vi "CSGaussmeter.setCTemp.vi"(0 "i ref in":refnum<vi>, 7 "CTemp":bool, 11 "error in (no error)":errorcluster) -> (4 "i ref out":refnum<vi>, 15 "error out":errorcluster)   [LabVIEW 2014, in "CSGaussmeter.lvlib"]
doc: "This VI sets the Temp. Correction ON or OFF. \n\nDurch dieses VI kann die Temperaturkorrektur an oder abgeschaltet werden. Die Temperaturkorrektur korrigiert die Temperaturabhängigkeit der Sondenempfindlichkeit und der Offsetspannung."
uses:
  CSGaussmeter.lvlib
  CS_Core/CSObj/CSObj.lvlib
  CSlibraries/UtilityLib/UtilityLib.lvlib
  instr.lib/FH_55/FH 55.lvlib
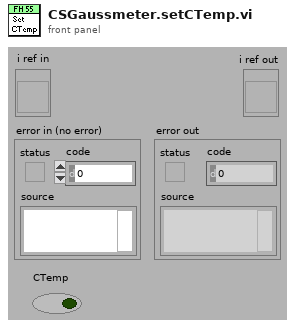
[diagram p1: front panel]
types:
  T1 = typedef "CSGaussmeter.lvlib/CSGaussmeter.i attribute.ctl" = cluster{"Name":string, "VISA Resource Name":refnum<visa-resource-name>, "actValues":cluster{" Limit":bool, "Unit ":T2, "Temp_Unit":T3, "Max":T4, " Filter":bool, " Peak":bool, " Auto_Range":bool, "Range":T5, " Rel":bool, " CTemp":bool, " CField":bool, "AC_DC ":bool, "Set_lower":cluster{"Numeric":dbl, "Cancel Button":bool, "Unit":T6}, "Set_upper":cluster{"Numeric":dbl, "Cancel Button":bool, "Unit":T6}, "Set_Rel":cluster{"Numeric":dbl, "Cancel Button":bool, "Unit":T6}, "Zero":bool, " Local":bool, "Reset":bool, " Init":bool}, "FH 55 Gauss-/Teslameter":T7, "MAX_Value":T8, "MIN_Value":T8, "Rel_Value":T8, "Array ":string[], "LIMU":dbl, " LIML":dbl, "Messwerte 2":string, "Messwerte ":cluster{"Numeric":i32, "OK Button":bool}, "serviceID":cluster{"Current ID":i32, "Unit ID":i32, "Temp ID":i32, "Name ID \n":i32, "Visa ID ":i32}, "setValues ":cluster{" Limit":bool, "Unit ":T2, "Temp_Unit":T3, "Max":T4, " Filter":bool, " Peak":bool, " Auto_Range":bool, "Range":T5, " Rel":bool, " CTemp":bool, " CField":bool, "AC_DC ":bool, "Set_lower":cluster{"Numeric":dbl, "Cancel Button":bool, "Unit":T6}, "Set_upper":cluster{"Numeric":dbl, "Cancel Button":bool, "Unit":T6}, "Set_Rel":cluster{"Numeric":dbl, "Cancel Button":bool, "Unit":T6}, "Zero":bool, " Local":bool, "Reset":bool, " Init":bool}}
  T2 = typedef "FH 55.lvlib/Unit.ctl" = enum16{"T", "G", "A/m"}
  T3 = typedef "FH 55.lvlib/Temp_Unit.ctl" = enum16{"Temp off", "Celsius", "Fahrenheit"}
  T4 = typedef "FH 55.lvlib/Max.ctl" = enum16{"MAX off", "Show MAX", "MAX/MIN"}
  T5 = typedef "FH 55.lvlib/Range.ctl" = enum16{"1", "2", "3", "4", "5", "6", "7"}
  T6 = typedef "FH 55.lvlib/Unit2.ctl" = enum16{"mT", "G", "kA/m"}
  T7 = typedef "FH 55.lvlib/Display.ctl" = cluster{"current value":string, "Limit":string, "Remote":string, "function ":string, "Cluster":cluster{"AC/DC":string, "Auto":string, "Filter":string, "Range":string, "Rel":string, "Peak":string}}
  T8 = typedef "FH 55.lvlib/Value_String.ctl" = cluster{"Numeric":dbl, "String":string}
  T9 = cluster{"VISA Resource Name":refnum<visa-resource-name>}
  T10 = typedef "FH 55.lvlib/VisaCluster.ctl" = cluster{"VISA Resource Name":refnum<visa-resource-name>}
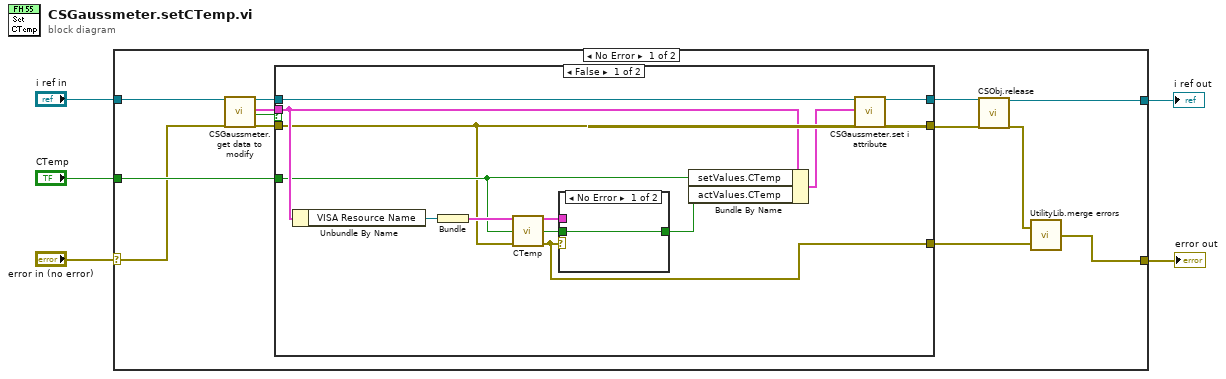
[diagram p0: block diagram]
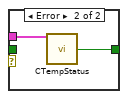
[diagram p2: hidden frame]
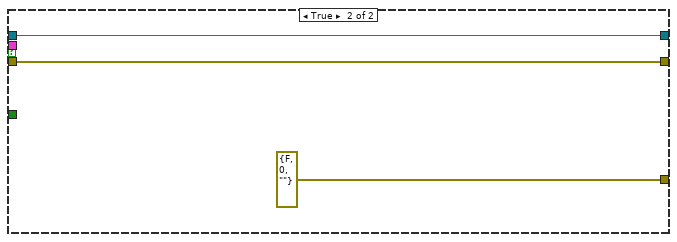
[diagram p3: hidden frame]
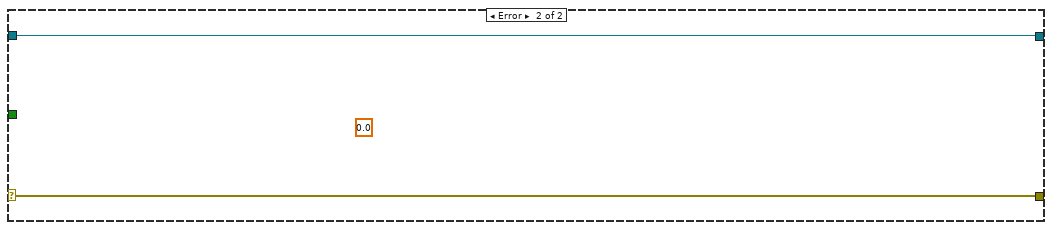
[diagram p4: hidden frame]
diagram:
  n1 = case shown="No Error" "error in (no error)" {
    selector: "error in (no error)" -> [w12 w38]
    tunnel: [w13 w38] -> w2
    tunnel: "i ref in" -> [w11 w39]
    tunnel: [w6 w39] -> w3
    tunnel: "CTemp" -> [w15 _]
    frame No Error {
      n2 = call "CSGaussmeter.get data to modify.vi"("i ref in"=w11, "error in (no error)"=w12) -> ("i ref out"=w10:refnum<vi>, "i attribute"=w9:T1, "timed out"=w8:bool, "error out"=w7:errorcluster)  [unwired: 14 in]
      n3 = case shown="False" w8 {
        tunnel: w10 -> [w29 w36]
        tunnel: w7 -> [w24 w37]
        tunnel: w9 -> [w30 _]
        tunnel: [w23 w37] -> w16
        tunnel: [w27 w36] -> w18
        tunnel: w15 -> [w25 _]
        tunnel: [w21 errorcluster {"status"=FALSE, "code"=0, "source"=""} ("error out")] -> w14
        frame False {
          n4 = Unbundle By Name(w30) -> ("VISA Resource Name"=w31:refnum<visa-resource-name>)
          n5 = Bundle("VISA Resource Name"=w31) -> (w26:T9)  [unwired: 1 in]
          n6 = call "CTemp.vi"("VisaCluster"=w26, "CTemp"=w25, "error in (no error)"=w24) -> ("VisaCluster"=w22:T10, "CTemp 2"=w20:bool, "error out"=w21:errorcluster)  [unwired: 9 in, 1 out]
          n7 = case shown="No Error" w21 {
            tunnel: w22 -> [_ w34]
            tunnel: w20 -> [w32 _]
            tunnel: [w32 w33] -> w19
            frame No Error {
            }
            frame Error {
              n8 = call "CTempStatus.vi"("VisaCluster"=w34) -> ("CTemp"=w33:bool)  [unwired: 11 in, 3 out]
            }
          }
          n9 = Bundle By Name(cluster=w30, "setValues.CTemp"=w25, "actValues.CTemp"=w19) -> (w28:T1)
          n10 = call "CSGaussmeter.set i attribute.vi"("i ref in"=w29, "i attribute"=w28, "error in (no error)"=w24) -> ("i ref out"=w27:refnum<vi>, "error out"=w23:errorcluster)  [unwired: 15 in]
        }
        frame True {
        }
      }
      n11 = call "CSObj.release.vi"("i ref in"=w18, "error in (no error)"=w16) -> ("i ref out"=w6:refnum<vi>, "error out"=w17:errorcluster)  [unwired: 16 in]
      n12 = call "UtilityLib.merge errors.vi"("error2 (no error)"=w14, "error1 (no error)"=w17) -> ("error out"=w13:errorcluster)
    }
    frame Error {
      (unwired) 0.0 ("Mid Setting [A or T]")
    }
  }
  "i ref out" <- w3
  "error out" <- w2
